vi "IOT sending data.vi"() -> ()   [LabVIEW 2018]
uses:
  <vilib>/httpClient/PUTBuffer.vi
  <vilib>/httpClient/LabVIEWHTTPClient.lvlib
panel:
  in  "?":dbl(knob) scale=0.0..10.0
  out "error out":errorcluster
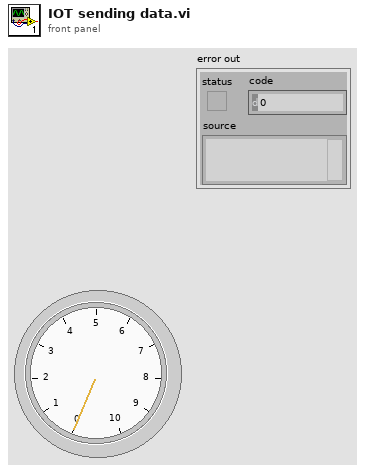
[diagram p1: front panel]
types:
  T1 = typedef "LabVIEWHTTPClient.lvlib/ClientHandle.ctl" = refnum<k1>
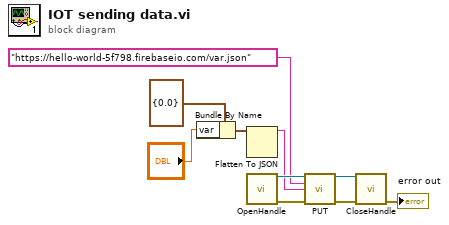
[diagram p0: block diagram]
diagram:
  n1 = Bundle By Name(cluster=cluster{"var":dbl} {"var"=0.0}, "var"="?") -> (w1:cluster{"var":dbl})
  n2 = Flatten To JSON(anything=w1) -> (JSON string=w4:string)  [unwired: 2 in, 1 out]
  n3 = call <vilib>:"OpenHandle.vi"() -> ("client handle out"=w10:T1, "error out"=w8:errorcluster)  [unwired: 14 in]
  n4 = call-poly <vilib>:"PUT.vi"("client handle"=w10, "url"="https://hello-world-5f798.firebaseio.com/var.json", "buffer"=w4, "error in (no error)"=w8) -> ("client handle out"=w9:T1, "error out"=w7:errorcluster)  [unwired: 8 in, 2 out]
  n5 = call <vilib>:"CloseHandle.vi"("client handle"=w9, "error in (no error)"=w7) -> ("error out"=→"error out":errorcluster)  [unwired: 13 in]
